vi "MatrixReset.vi"(8 "error in (no error)":errorcluster, 11 "KE3700A in":refnum<class "KE3706A.lvclass">) -> (0 "error out":errorcluster, 3 "KE3700A out":refnum<class "KE3706A.lvclass">)   [LabVIEW 2013, in "KE3706A.lvclass"]
uses:
  KE3706A.lvclass
  <instrlib>/Keithley 3706/Keithley 3700 Series.lvlib
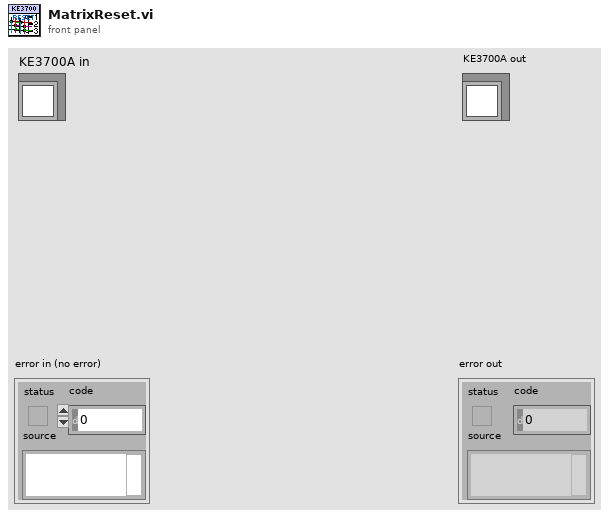
[diagram p1: front panel]
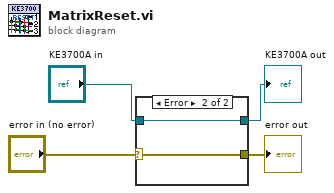
[diagram p0: block diagram]
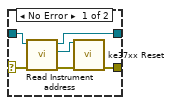
[diagram p2: hidden frame]
diagram:
  n1 = case shown="Error" "error in (no error)" {
    selector: "error in (no error)" -> [w8 w12]
    tunnel: [w5 w12] -> w3
    tunnel: "KE3700A in" -> [w10 w11]
    tunnel: [w9 w11] -> w1
    frame No Error {
      n2 = call-dynamic "Read Instrument address.vi"("error in (no error)"=w8, "InstControl in"=w10) -> ("error out"=w7:errorcluster, "VISA address"=w6:refnum<visa-resource-name>, "InstControl out"=w9:refnum<class "KE3706A.lvclass">)  [unwired: 7 in]
      n3 = call <instrlib>:"ke37xx Reset.vi"("VISA resource name"=w6, "error in (no error)"=w7) -> ("error out"=w5:errorcluster)  [unwired: 12 in, 1 out]
    }
    frame Error {
    }
  }
  "error out" <- w3
  "KE3700A out" <- w1
